vi "lorentzian from circle corners V6.vi"(6 "fragment  : cursor window":T4={"left"=2378.60310421286, "right "=2421.6740576496672, "center"=2421.6740576496672, "window"=2421.6740576496672, "cursors"=[], "relative"=0, "absolute"=0, "plot ref"=refnum, "Cursor List"=[], "fixed vertical offset"=2421.6740576496672, "vertical offset"=2421.6740576496672, "horizontal offset"=2421.6740576496672, "default window frac"=2421.6740576496672, "kind"=enum."symmetric"}, 7 "update z(inf)":enum16{"update z(inf)", "do not update z(inf)"}(ring)=enum."do not update z(inf)", 8 "omega map rameters in":T6={"map method"=enum."less trivial", "2:window factor"=1, "left"=3.0, "right"=3.0, "omega"=3.0, "gamma"=3.0, "theta0"=3.0, "use points"=enum."decimated", "z(inf) method"=enum."median"}, 9 "main VI  path":path, 10 "parameters in: center detection":T3={"number of 2D grid points"=200, "# of points in pond"=93, "# of points in window"=4107, "decimation threshold"=1, "normalization factor"=0.005102552585135461, "pond scale factor "=3.0, "normalized z"=[], "decimated z"=[], "decimated omega"=[], "omega in window"=[], "z in window"=[], "data center"=-0.0014901433980738042-0.0014987103874714112i, "inverse"=[], "linear "=[], "omega around"=[], "phase around center"=[], "fit for phase around senter "=[], "three points"={[], []}}, 11 "lorentzian in":T1={"Amplitude"=-1.0311345636926572, "omega(0)"=-1.0311345636926572, "Gamma"=-1.0311345636926572, "phase"=-1.0311345636926572, "Q"=-1.0311345636926572, "Norm  Ampl"=-1.0311345636926572, "z (inf)"=-1.0311345636926572+0.0i, "4corners"={"z (-pi/2)"=-1.0311345636926572+0.5736824521422934i, "z(inf)"=-0.5200164984937075+1.0975277942502903i, "z (pi/2)"=-1.0311345636926572+0.5736824521422934i, "z center"=-0.5136528600391839+0.580046090596817i, "z(0)"=-0.5200164984937075+1.0975277942502903i, "radius"=-1.0311345636926572}} {"Q" format="%#_8f"; "phase" format="%#_6f"; "Gamma" format="%#_8f"; "omega(0)" format="%#_8f"}) -> (0 "omega map parameters  out":T6={"map method"=enum."less trivial", "2:window factor"=1, "left"=3.0, "right"=3.0, "omega"=3.0, "gamma"=3.0, "theta0"=3.0, "use points"=enum."decimated", "z(inf) method"=enum."median"}, 2 "parameters out  : center detection":T3={"number of 2D grid points"=200, "# of points in pond"=93, "# of points in window"=4107, "decimation threshold"=1, "normalization factor"=0.005102552585135461, "pond scale factor "=3.0, "normalized z"=[], "decimated z"=[], "decimated omega"=[], "omega in window"=[], "z in window"=[], "data center"=-0.0014901433980738042-0.0014987103874714112i, "inverse"=[], "linear "=[], "omega around"=[], "phase around center"=[], "fit for phase around senter "=[], "three points"={[], []}}, 3 "lorentzian out":T1={"Amplitude"=-1.0311345636926572, "omega(0)"=-1.0311345636926572, "Gamma"=-1.0311345636926572, "phase"=-1.0311345636926572, "Q"=-1.0311345636926572, "Norm  Ampl"=-1.0311345636926572, "z (inf)"=-1.0311345636926572+0.0i, "4corners"={"z (-pi/2)"=-1.0311345636926572+0.5736824521422934i, "z(inf)"=-0.5200164984937075+1.0975277942502903i, "z (pi/2)"=-1.0311345636926572+0.5736824521422934i, "z center"=-0.5136528600391839+0.580046090596817i, "z(0)"=-0.5200164984937075+1.0975277942502903i, "radius"=-1.0311345636926572}} {"Q" format="%#_8f"; "phase" format="%#_6f"; "Gamma" format="%#_8f"; "omega(0)" format="%#_8f"})   [LabVIEW 2010]
uses:
  lorentzian.ctl
  circle corners.ctl
  omega map parameters.ctl
  single fit parameters.ctl
  cursor winow.ctl
  <vilib>/Utility/miscctls.llb/LVCursorListTypeDef.ctl
  <vilib>/gmath/NumericalOptimization/LM model function reference.ctl
  <vilib>/Analysis/6fits.llb/Curve Fitting Criteria.ctl
  <vilib>/Analysis/baseanly.llb/Mean.vi
  <vilib>/Analysis/baseanly.llb/Median.vi
  <vilib>/gmath/NumericalOptimization/Nonlinear Curve Fit LM.vi
  <vilib>/Analysis/NI_AALPro.lvlib
  <vilib>/gmath/NI_Gmath.lvlib
  <vilib>/gmath/NumericalOptimization/Nonlinear Curve Fit LM formula string.vi
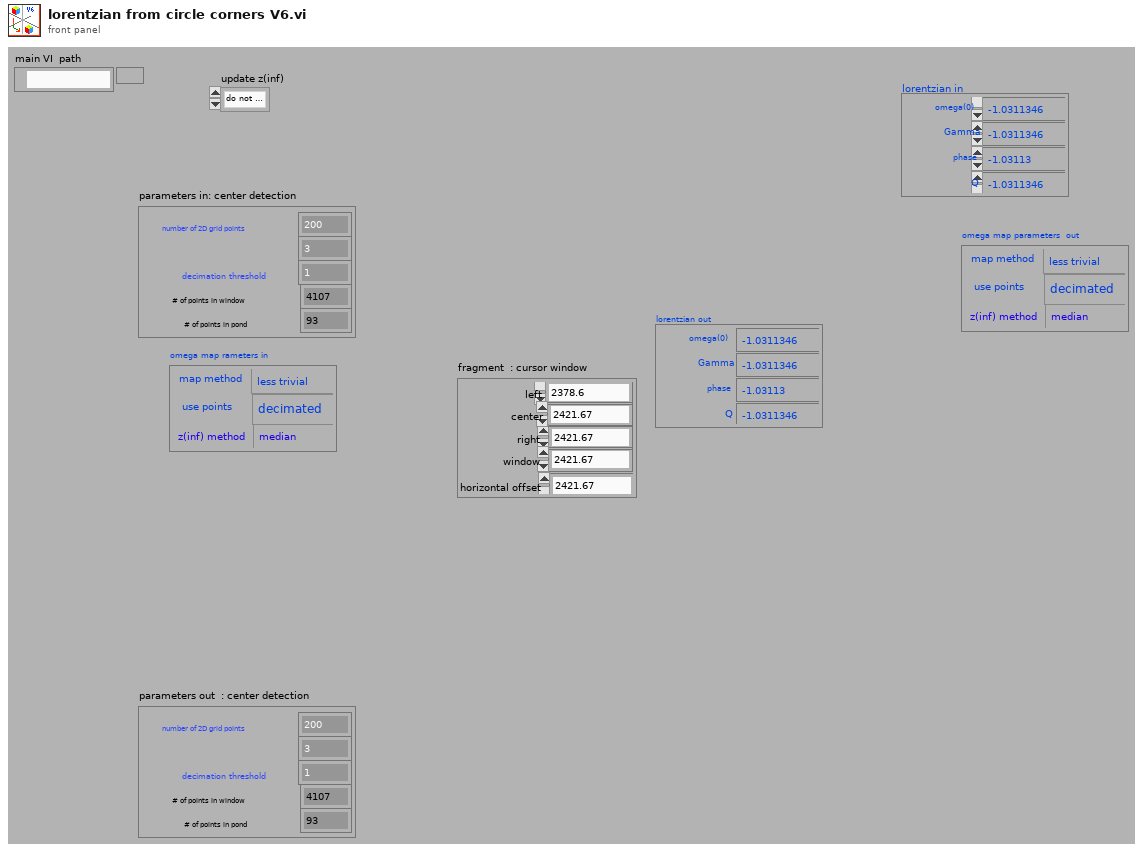
[diagram p1: front panel]
types:
  T1 = typedef "lorentzian.ctl" = cluster{"Amplitude":dbl, "omega(0)":dbl, "Gamma":dbl, "phase":dbl, "Q":dbl, "Norm  Ampl":dbl, "z (inf)":cdb, "4corners":T2}
  T2 = typedef "circle corners.ctl" = cluster{"z (-pi/2)":cdb, "z(inf)":cdb, "z (pi/2)":cdb, "z center":cdb, "z(0)":cdb, "radius":dbl}
  T3 = typedef "single fit parameters.ctl" = cluster{"number of 2D grid points":i32, "# of points in pond":i32, "# of points in window":i32, "decimation threshold":i32, "normalization factor":dbl, "pond scale factor ":dbl, "normalized z":cdb[], "decimated z":cdb[], "decimated omega":dbl[], "omega in window":dbl[], "z in window":cdb[], "data center":cdb, "inverse":cdb[], "linear ":cdb[], "omega around":dbl[], "phase around center":dbl[], "fit for phase around senter ":dbl[], "three points":cluster{dbl[], dbl[]}}
  T4 = typedef "cursor winow.ctl" = cluster{"left":dbl, "right ":dbl, "center":dbl, "window":dbl, "cursors":i32[], "relative":i32, "absolute":i32, "plot ref":refnum<vi>, "Cursor List":T5, "fixed vertical offset":dbl, "vertical offset":dbl, "horizontal offset":dbl, "default window frac":dbl, "kind":enum16{"symmetric", "skewed", "fancy"}}
  T5 = typedef "LVCursorListTypeDef.ctl" = cluster{"Name":string, "Color":u32, "Style":u8, "Point Style":u8, "Name Visible":bool, "Allow Drag":bool, "Cursor Mode":u32, "Plot":i32, "Index":i32, "Position":cluster{"X":dbl, "Y":dbl}, "X Scale":u32, "Y Scale":u32, "Watch Plots":i32[], "Watch All Plots":bool, "Plot Area":i32, "Label Offset":cluster{"X":dbl, "Y":dbl}}[]
  T6 = typedef "omega map parameters.ctl" = cluster{"map method":enum16{"simple", "less trivial", "around center", "geometry"}, "2:window factor":i32, "left":dbl, "right":dbl, "omega":dbl, "gamma":dbl, "theta0":dbl, "use points":enum16{"all in window", "decimated"}, "z(inf) method":enum16{"median", "method 2", "histogram"}}
  T7 = enum16{"simple", "less trivial", "around center", "geometry"}
  T8 = typedef "NI_Gmath.lvlib/LM model function reference.ctl" = refnum<vi>
  T9 = cluster{"model":string, "Parameters":string[], "x":string}
  T10 = typedef "NI_AALPro.lvlib/Curve Fitting Criteria.ctl" = u16
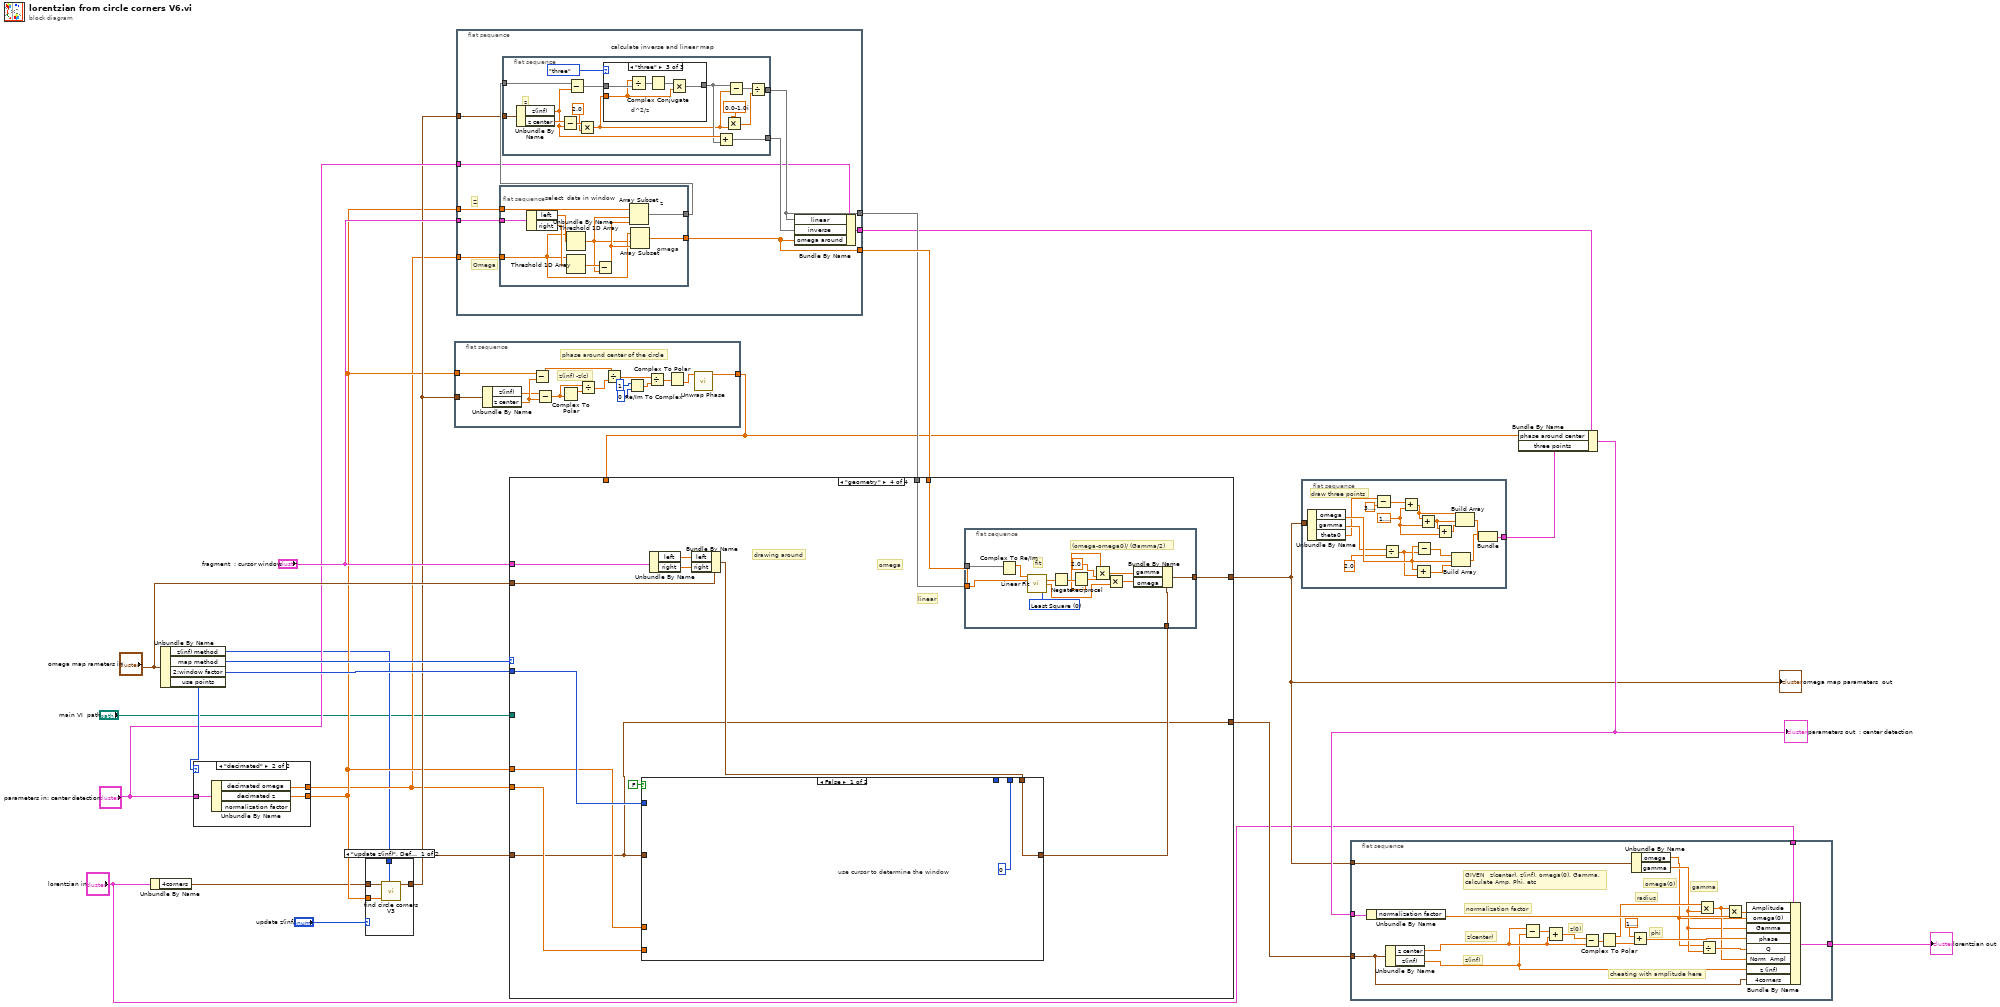
[diagram p0: block diagram]
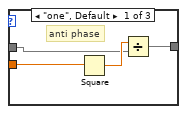
[diagram p2: hidden frame]
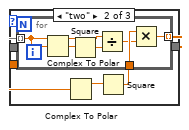
[diagram p3: hidden frame]
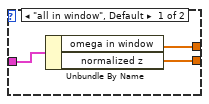
[diagram p5: hidden frame]
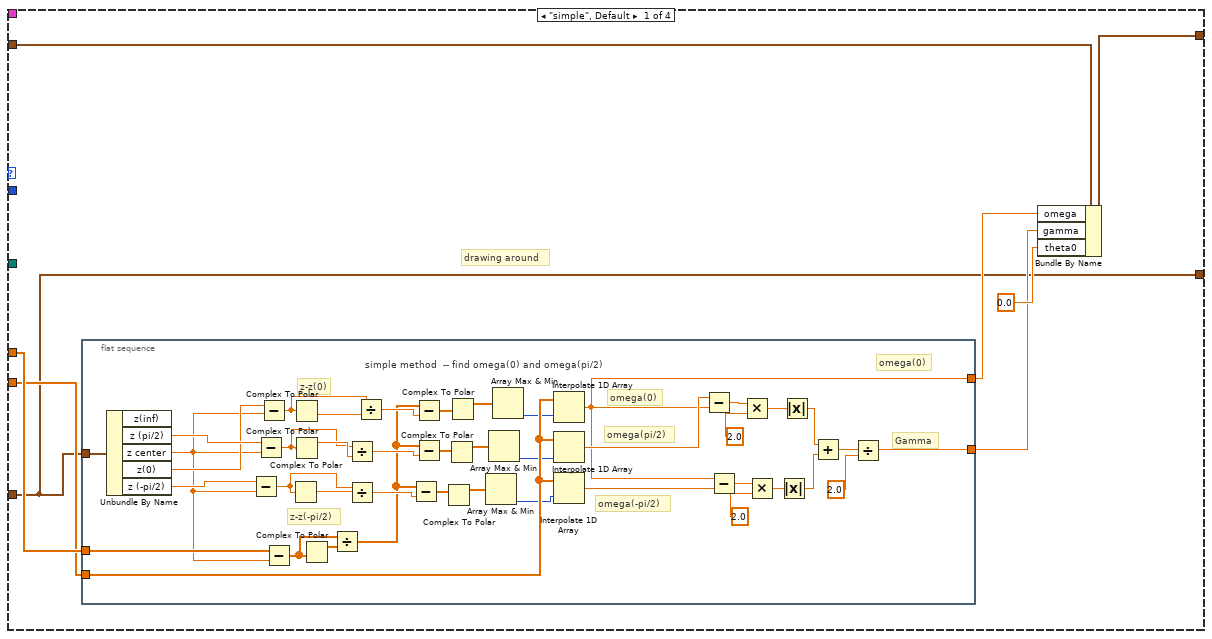
[diagram p6: hidden frame]
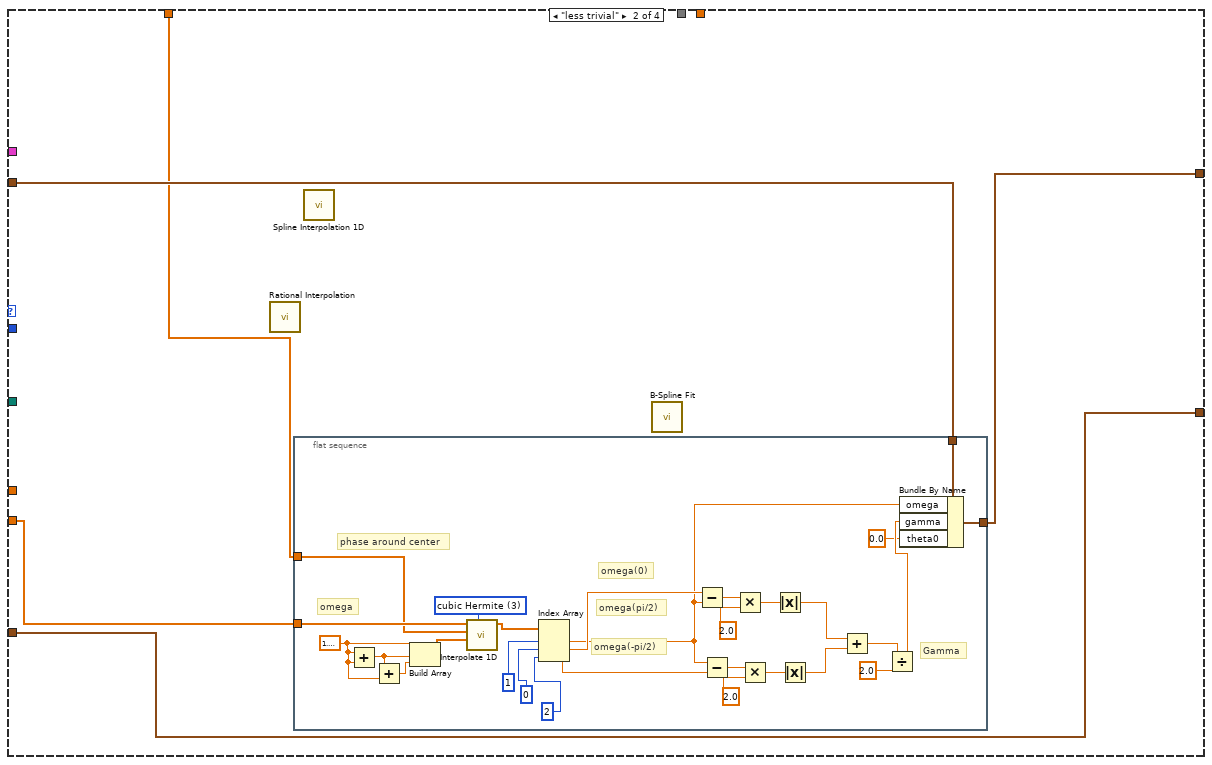
[diagram p7: hidden frame]
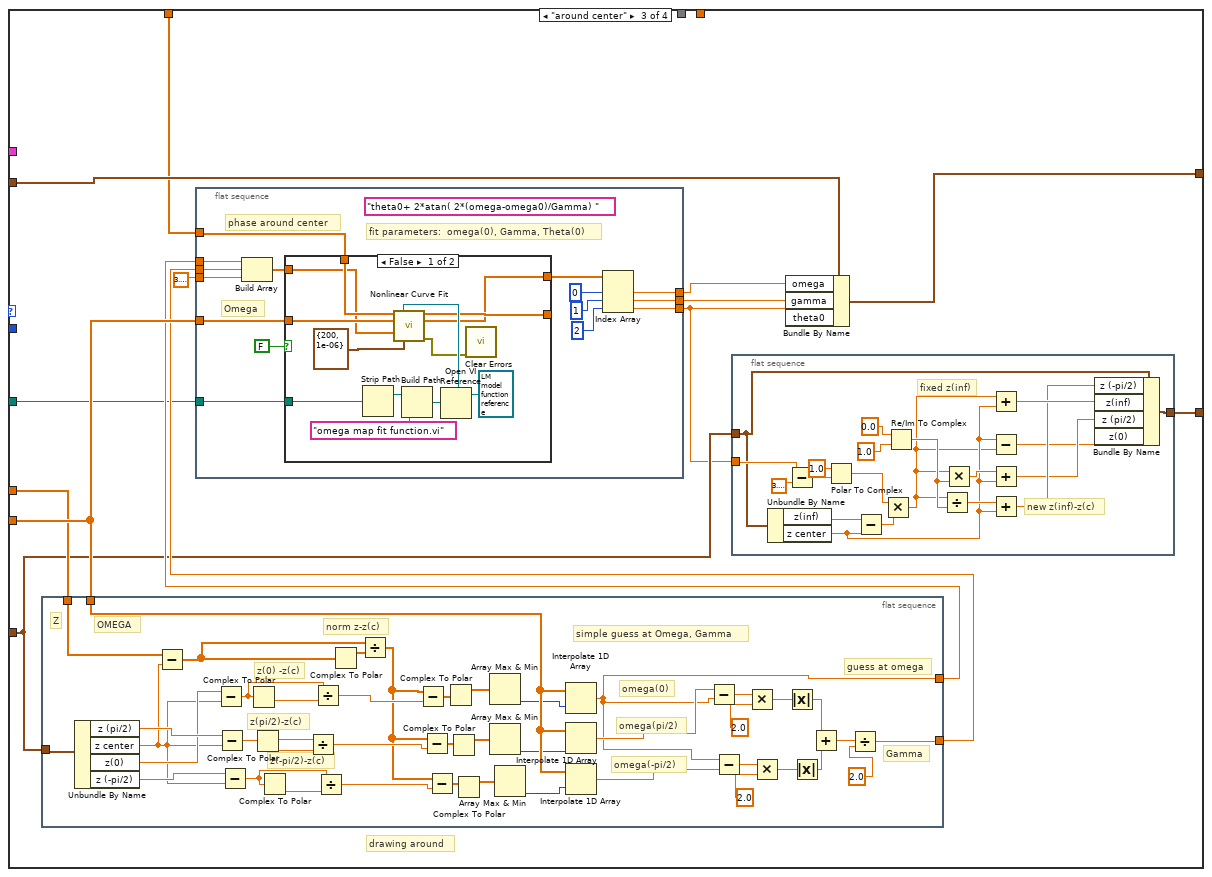
[diagram p8: hidden frame]
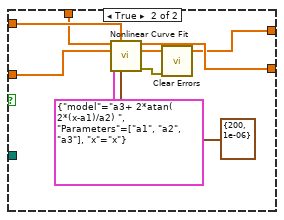
[diagram p9: hidden frame]
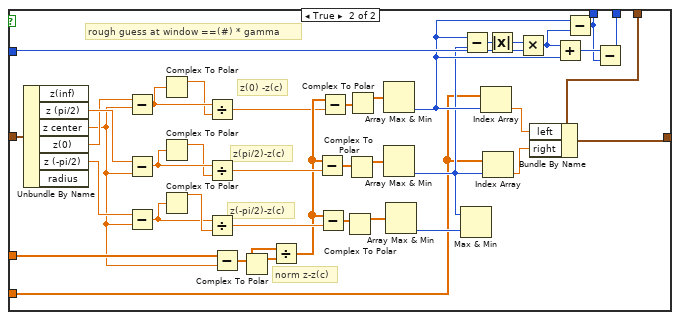
[diagram p10: hidden frame]
diagram:
  n1 = Unbundle By Name("lorentzian in") -> ("4corners"=w3:T2)
  n2 = Unbundle By Name("omega map rameters in") -> ("z(inf) method"=w4:enum16{"median", "method 2", "histogram"}, "map method"=w23:T7, "2:window factor"=w21:i32, "use points"=w20:enum16{"all in window", "decimated"})
  n3 = case shown="\"decimated\"" w20 {
    tunnel: "parameters in: center detection" -> [w26 w29]
    tunnel: [w25 w28] -> w11
    tunnel: [w24 w27] -> w13
    frame "all in window", Default {
      n4 = Unbundle By Name(w26) -> ("omega in window"=w25:dbl[], "normalized z"=w24:cdb[])
    }
    frame "decimated" {
      n5 = Unbundle By Name(w29) -> ("decimated omega"=w28:dbl[], "decimated z"=w27:cdb[])  [unwired: 1 out]
    }
  }
  n6 = case shown="\"update z(inf)\", Default" "update z(inf)" {
    tunnel: [w32 w34] -> w14
    tunnel: w3 -> [w33 w34]
    tunnel: w13 -> [w31 _]
    tunnel: w4 -> [w30 _]
    frame "update z(inf)", Default {
      n7 = call "find circle corners V3.vi"("method"=w30, "z"=w31, "circle corners in"=w33) -> ("circle corners out"=w32:T2)  [unwired: 8 in]
    }
    frame "do not update z(inf)" {
    }
  }
  n8 = flat-sequence {
    tunnel: w14 -> [w37]
    tunnel: w13 -> [w36]
    tunnel: [w35] -> w9
    frame #0 {
      # "phase around center of the circle"
      # "z(inf) -z(c)"
      n9 = Unbundle By Name(w37) -> ("z(inf)"=w39:cdb, "z center"=w40:cdb)
      n10 = Subtract(x=w36, y=w40) -> (x-y=w48:cdb[])
      n11 = Subtract(x=w39, y=w40) -> (x-y=w38:cdb)
      n12 = Complex To Polar(r * e^(i*theta)=w38) -> (r=w49:dbl)  [unwired: 1 out]
      n13 = Divide(x=w38, y=w49) -> (x/y=w41:cdb)
      n14 = Divide(x=w48, y=w41) -> (x/y=w44:cdb[])
      n15 = Re/Im To Complex(1:0, 2:1) -> (0:w46:cdb)
      n16 = Divide(x=w44, y=w46) -> (x/y=w47:cdb[])
      n17 = Complex To Polar(r * e^(i*theta)=w47) -> (theta=w42:dbl[])  [unwired: 1 out]
      n18 = call <vilib>:"Unwrap Phase.vi"("Phase"=w42) -> ("Unwrapped Phase"=w35:dbl[])  [unwired: 9 in, 1 out]
    }
  }
  n19 = flat-sequence {
    tunnel: [w57] -> w18
    tunnel: w14 -> [w56]
    tunnel: w13 -> [w55]
    tunnel: "fragment  : cursor window" -> [w54]
    tunnel: w11 -> [w53]
    tunnel: [w52] -> w10
    tunnel: [w51] -> w16
    tunnel: "parameters in: center detection" -> [w50]
    frame #0 {
      # "calculate inverse and linear map"
      # "Z"
      # "Omega"
      n20 = flat-sequence {
        tunnel: [w100] -> w58
        tunnel: [w99] -> w57
        tunnel: w55 -> [w98]
        tunnel: w54 -> [w97]
        tunnel: w53 -> [w96]
        frame #0 {
          # "select  data in window"
          # "omega"
          # "z"
          n21 = Unbundle By Name(w97) -> ("left"=w101:dbl, "right"=w102:dbl)
          n22 = Threshold 1D Array(2:w101, 3:w96) -> (0:w95:dbl)  [unwired: 1 in]
          n23 = Threshold 1D Array(2:w102, 3:w96) -> (0:w103:dbl)  [unwired: 1 in]
          n24 = Subtract(x=w103, y=w95) -> (x-y=w104:dbl)
          n25 = Array Subset(array=w98, index=w95, length=w104) -> (w100:cdb[])
          n26 = Array Subset(array=w96, index=w95, length=w104) -> (w99:dbl[])
        }
      }
      n27 = flat-sequence {
        tunnel: [w74] -> w59
        tunnel: w58 -> [w69]
        tunnel: w56 -> [w63]
        tunnel: [w62] -> w51
        frame #0 {
          # "z"
          n28 = Unbundle By Name(w63) -> ("z(inf)"=w72:cdb, "z center"=w73:cdb)
          n29 = Subtract(x=w73, y=w72) -> (x-y=w65:cdb)
          n30 = Subtract(x=w69, y=w72) -> (x-y=w66:cdb[])
          n31 = Multiply(x=w65, y=2.0) -> (x*y=w61:cdb)
          n32 = case shown="\"three\"" enum16{"one", "three", "two"}."three" {
            tunnel: w66 -> [w76 w83 w94]
            tunnel: [w75 w80 w90] -> w67
            tunnel: w61 -> [w78 w79 w91]
            frame "one", Default {
              # "anti phase"
              n33 = Square(x=w78) -> (x^2=w77:cdb)
              n34 = Divide(x=w77, y=w76) -> (x/y=w75:cdb[])
            }
            frame "two" {
              n35 = Complex To Polar(r * e^(i*theta)=w79) -> (r=w82:dbl)  [unwired: 1 out]
              n36 = Square(x=w82) -> (x^2=w81:dbl)
              n37 = for {
                tunnel: w83 -> [w89] mode=indexing
                tunnel: w81 -> [w86]
                tunnel: [w84] -> w80 mode=indexing
                n38 = Complex To Polar(r * e^(i*theta)=w89) -> (r=w87:dbl)  [unwired: 1 out]
                n39 = Square(x=w87) -> (x^2=w88:dbl)
                n40 = Divide(x=w89, y=w88) -> (x/y=w85:cdb)
                n41 = Multiply(x=w86, y=w85) -> (x*y=w84:cdb)
              }
            }
            frame "three" {
              # "d^2/z"
              n42 = Divide(x=w91, y=w94) -> (x/y=w93:cdb[])
              n43 = Complex Conjugate(1:w93) -> (0:w92:cdb[])
              n44 = Multiply(x=w92, y=w91) -> (x*y=w90:cdb[])
            }
          }
          n45 = Add(x=w72, y=w67) -> (x+y=w74:cdb[])
          n46 = Multiply(x=cdb 0.0-1.0i ("y"), y=w61) -> (x*y=w70:cdb)
          n47 = Subtract(x=w67, y=w61) -> (x-y=w68:cdb[])
          n48 = Divide(x=w68, y=w70) -> (x/y=w62:cdb[])
        }
      }
      n49 = Bundle By Name(cluster=w50, "linear"=w51, "inverse"=w59, "omega around"=w57) -> (w52:T3)
    }
  }
  n50 = case shown="\"geometry\"" w23 {
    tunnel: w14 -> [w105 w155 w192 w300]
    tunnel: w13 -> [w112 _ w193 w311]
    tunnel: w11 -> [w111 w157 w200 w302]
    tunnel: "omega map rameters in" -> [w109 w159 w199 w309]
    tunnel: [w108 w158 w201 w313] -> w6
    tunnel: w21 -> [_ _ _ w312]
    tunnel: "fragment  : cursor window" -> [_ _ _ w304]
    tunnel: w18 -> [_ _ _ w303]
    tunnel: w16 -> [_ _ _ w301]
    tunnel: w9 -> [_ w156 w191 _]
    tunnel: [w105 w155 w189 w300] -> w5
    tunnel: "main VI  path" -> [_ _ w188 _]
    frame "simple", Default {
      # "drawing around"
      n51 = flat-sequence {
        tunnel: w105 -> [w150]
        tunnel: w112 -> [w149]
        tunnel: w111 -> [w138]
        tunnel: [w115] -> w107
        tunnel: [w114] -> w106
        frame #0 {
          # "simple method  -- find omega(0) and omega(pi/2)"
          # "omega(0)"
          # "z-z(-pi/2)"
          # "z-z(0)"
          # "omega(-pi/2)"
          # "omega(pi/2)"
          # "omega(0)"
          # "Gamma"
          n52 = Unbundle By Name(w150) -> ("z (pi/2)"=w148:cdb, "z center"=w113:cdb, "z(0)"=w147:cdb, "z (-pi/2)"=w146:cdb)  [unwired: 1 out]
          n53 = Subtract(x=w146, y=w113) -> (x-y=w133:cdb)
          n54 = Subtract(x=w148, y=w113) -> (x-y=w132:cdb)
          n55 = Subtract(x=w147, y=w113) -> (x-y=w137:cdb)
          n56 = Subtract(x=w149, y=w113) -> (x-y=w130:cdb[])
          n57 = Complex To Polar(r * e^(i*theta)=w133) -> (r=w135:dbl)  [unwired: 1 out]
          n58 = Complex To Polar(r * e^(i*theta)=w137) -> (r=w136:dbl)  [unwired: 1 out]
          n59 = Complex To Polar(r * e^(i*theta)=w132) -> (r=w134:dbl)  [unwired: 1 out]
          n60 = Complex To Polar(r * e^(i*theta)=w130) -> (r=w131:dbl[])  [unwired: 1 out]
          n61 = Divide(x=w130, y=w131) -> (x/y=w126:cdb[])
          n62 = Divide(x=w132, y=w134) -> (x/y=w128:cdb)
          n63 = Divide(x=w133, y=w135) -> (x/y=w127:cdb)
          n64 = Divide(x=w137, y=w136) -> (x/y=w129:cdb)
          n65 = Subtract(x=w126, y=w127) -> (x-y=w124:cdb[])
          n66 = Subtract(x=w126, y=w129) -> (x-y=w125:cdb[])
          n67 = Subtract(x=w126, y=w128) -> (x-y=w123:cdb[])
          n68 = Complex To Polar(r * e^(i*theta)=w124) -> (r=w120:dbl[])  [unwired: 1 out]
          n69 = Complex To Polar(r * e^(i*theta)=w123) -> (r=w121:dbl[])  [unwired: 1 out]
          n70 = Complex To Polar(r * e^(i*theta)=w125) -> (r=w122:dbl[])  [unwired: 1 out]
          n71 = Array Max & Min(array=w120) -> (min index (indices)=w119:i32)  [unwired: 3 out]
          n72 = Array Max & Min(array=w121) -> (min index (indices)=w118:i32)  [unwired: 3 out]
          n73 = Array Max & Min(array=w122) -> (min index (indices)=w117:i32)  [unwired: 3 out]
          n74 = Interpolate 1D Array(1:w117, 2:w138) -> (0:w115:dbl)
          n75 = Interpolate 1D Array(1:w118, 2:w138) -> (0:w151:dbl)
          n76 = Interpolate 1D Array(1:w119, 2:w138) -> (0:w139:dbl)
          n77 = Subtract(x=w151, y=w115) -> (x-y=w154:dbl)
          n78 = Subtract(x=w115, y=w139) -> (x-y=w145:dbl)
          n79 = Multiply(x=w154, y=2.0) -> (x*y=w152:dbl)
          n80 = Multiply(x=w145, y=2.0) -> (x*y=w143:dbl)
          n81 = Absolute Value(x=w143) -> (abs(x)=w116:dbl)
          n82 = Absolute Value(x=w152) -> (abs(x)=w142:dbl)
          n83 = Add(x=w142, y=w116) -> (x+y=w141:dbl)
          n84 = Divide(x=w141, y=2.0) -> (x/y=w114:dbl)
        }
      }
      n85 = Bundle By Name(cluster=w109, "omega"=w107, "gamma"=w106, "theta0"=0.0 ("phi0")) -> (w108:T6)
    }
    frame "less trivial" {
      n86 = call <vilib>:"Rational Interpolation.vi"() -> ()  [unwired: 3 in, 3 out]
      n87 = flat-sequence {
        tunnel: w159 -> [w166]
        tunnel: [w165] -> w158
        tunnel: w157 -> [w162]
        tunnel: w156 -> [w161]
        frame #0 {
          w175 = 1.5707963267948966
          w177 = 3 items=["nearest", "linear", "spline", "cubic Hermite", "Lagrange"] ("method")
          # "phase around center"
          # "omega"
          # "omega(-pi/2)"
          # "omega(pi/2)"
          # "omega(0)"
          # "Gamma"
          n88 = Add(x=w175, y=w175) -> (x+y=w176:dbl)
          n89 = Add(x=w176, y=w175) -> (x+y=w174:dbl)
          n90 = Build Array(w175, w176, w174) -> (w173:dbl[])
          n91 = call <vilib>:"Interpolate 1D.vi"("method"=w177, "xi"=w173, "X"=w161, "Y"=w162) -> ("yi"=w169:dbl[])  [unwired: 5 in, 2 out]
          n92 = Index Array(array=w169, index #1=1, index #2=0, index #3=2) -> (element #1=w164:dbl, element #2=w168:dbl, element #3=w167:dbl)
          n93 = Subtract(x=w168, y=w164) -> (x-y=w187:dbl)
          n94 = Subtract(x=w164, y=w167) -> (x-y=w184:dbl)
          n95 = Multiply(x=w187, y=2.0) -> (x*y=w185:dbl)
          n96 = Multiply(x=w184, y=2.0) -> (x*y=w182:dbl)
          n97 = Absolute Value(x=w185) -> (abs(x)=w181:dbl)
          n98 = Absolute Value(x=w182) -> (abs(x)=w178:dbl)
          n99 = Add(x=w181, y=w178) -> (x+y=w180:dbl)
          n100 = Divide(x=w180, y=2.0) -> (x/y=w163:dbl)
          n101 = Bundle By Name(cluster=w166, "omega"=w164, "gamma"=w163, "theta0"=0.0 ("phi0")) -> (w165:T6)
        }
      }
      n102 = call <vilib>:"Spline Interpolation 1D.vi"() -> ()  [unwired: 9 in, 3 out]
      n103 = call <vilib>:"B-Spline Fit.vi"() -> ()  [unwired: 12 in, 4 out]
    }
    frame "around center" {
      # "drawing around"
      n104 = flat-sequence {
        tunnel: w200 -> [w299]
        tunnel: [w267] -> w195
        tunnel: [w264] -> w194
        tunnel: w192 -> [w263]
        tunnel: w193 -> [w261]
        frame #0 {
          # "guess at omega"
          # "simple guess at Omega, Gamma"
          # "OMEGA"
          # "Z"
          # "norm z-z(c)"
          # "omega(-pi/2)"
          # "omega(pi/2)"
          # "omega(0)"
          # "Gamma"
          # "z(pi/2)-z(c)"
          # "z(-pi/2)-z(c)"
          # "z(0) -z(c)"
          n105 = Unbundle By Name(w263) -> ("z (pi/2)"=w298:cdb, "z center"=w262:cdb, "z(0)"=w297:cdb, "z (-pi/2)"=w296:cdb)
          n106 = Subtract(x=w261, y=w262) -> (x-y=w259:cdb[])
          n107 = Subtract(x=w297, y=w262) -> (x-y=w295:cdb)
          n108 = Subtract(x=w298, y=w262) -> (x-y=w291:cdb)
          n109 = Subtract(x=w296, y=w262) -> (x-y=w292:cdb)
          n110 = Complex To Polar(r * e^(i*theta)=w295) -> (r=w294:dbl)  [unwired: 1 out]
          n111 = Complex To Polar(r * e^(i*theta)=w291) -> (r=w281:dbl)  [unwired: 1 out]
          n112 = Complex To Polar(r * e^(i*theta)=w292) -> (r=w293:dbl)  [unwired: 1 out]
          n113 = Divide(x=w291, y=w281) -> (x/y=w289:cdb)
          n114 = Divide(x=w295, y=w294) -> (x/y=w290:cdb)
          n115 = Divide(x=w292, y=w293) -> (x/y=w288:cdb)
          n116 = Complex To Polar(r * e^(i*theta)=w259) -> (r=w260:dbl[])  [unwired: 1 out]
          n117 = Divide(x=w259, y=w260) -> (x/y=w258:cdb[])
          n118 = Subtract(x=w258, y=w290) -> (x-y=w287:cdb[])
          n119 = Subtract(x=w258, y=w289) -> (x-y=w285:cdb[])
          n120 = Subtract(x=w258, y=w288) -> (x-y=w286:cdb[])
          n121 = Complex To Polar(r * e^(i*theta)=w287) -> (r=w284:dbl[])  [unwired: 1 out]
          n122 = Complex To Polar(r * e^(i*theta)=w285) -> (r=w283:dbl[])  [unwired: 1 out]
          n123 = Complex To Polar(r * e^(i*theta)=w286) -> (r=w282:dbl[])  [unwired: 1 out]
          n124 = Array Max & Min(array=w284) -> (min index (indices)=w270:i32)  [unwired: 3 out]
          n125 = Array Max & Min(array=w283) -> (min index (indices)=w269:i32)  [unwired: 3 out]
          n126 = Array Max & Min(array=w282) -> (min index (indices)=w268:i32)  [unwired: 3 out]
          n127 = Interpolate 1D Array(1:w270, 2:w299) -> (0:w264:dbl)
          n128 = Interpolate 1D Array(1:w269, 2:w299) -> (0:w266:dbl)
          n129 = Interpolate 1D Array(1:w268, 2:w299) -> (0:w265:dbl)
          n130 = Subtract(x=w266, y=w264) -> (x-y=w280:dbl)
          n131 = Subtract(x=w264, y=w265) -> (x-y=w277:dbl)
          n132 = Multiply(x=w280, y=2.0) -> (x*y=w278:dbl)
          n133 = Multiply(x=w277, y=2.0) -> (x*y=w275:dbl)
          n134 = Absolute Value(x=w278) -> (abs(x)=w274:dbl)
          n135 = Absolute Value(x=w275) -> (abs(x)=w271:dbl)
          n136 = Add(x=w274, y=w271) -> (x+y=w273:dbl)
          n137 = Divide(x=w273, y=2.0) -> (x/y=w267:dbl)
        }
      }
      n138 = flat-sequence {
        tunnel: w200 -> [w236]
        tunnel: [w235] -> w198
        tunnel: [w234] -> w197
        tunnel: 3.141592653589793 -> [w233]
        tunnel: w195 -> [w231]
        tunnel: w194 -> [w230]
        tunnel: [w225] -> w190
        tunnel: w191 -> [w223]
        tunnel: w188 -> [w222]
        frame #0 {
          (unwired) "theta0+ 2*atan( 2*(omega-omega0)/Gamma) " ("model")
          # "phase around center"
          # "Omega"
          # "fit parameters:  omega(0), Gamma, Theta(0)"
          n139 = Build Array(w230, w231, w233) -> (w232:dbl[])
          n140 = case shown="False" FALSE {
            tunnel: w236 -> [w241 w257]
            tunnel: w232 -> [w240 w256]
            tunnel: [w239 w255] -> _
            tunnel: w223 -> [w242 w254]
            tunnel: [w238 w253] -> w229
            tunnel: w222 -> [w237 _]
            frame False {
              n141 = Strip Path(path=w237) -> (stripped path=w248:path)  [unwired: 1 out]
              n142 = Build Path(base path=w248, name or relative path="omega map fit function.vi" ("f(x,a) VI name Complex")) -> (appended path=w246:path)
              n143 = Open VI Reference(type specifier VI Refnum (for type only)=T8 refnum ("f(x,a)"), vi path=w246) -> (vi reference=w245:T8)  [unwired: 1 in, 4 out]
              n144 = call-poly <vilib>:"Nonlinear Curve Fit.vi"("Y"=w242, "f(x,a)"=w245, "X"=w241, "initial parameters"=w240, "termination"=cluster{"max iteration":i32, "tolerance":dbl} {"max iteration"=200, "tolerance"=1e-06}) -> ("best nonlinear fit"=w239:dbl[], "best fit parameters"=w238:dbl[], "error out"=w243:errorcluster)  [unwired: 5 in, 3 out]
              n145 = call <vilib>:"Clear Errors.vi"("error in (no error)"=w243) -> ()  [unwired: 6 in, 1 out]
            }
            frame True {
              n146 = call-poly <vilib>:"Nonlinear Curve Fit.vi"("Y"=w254, "initial parameters"=w256, "X"=w257, "model description"=T9 {"model"="a3+ 2*atan( 2*(x-a1)/a2) ", "Parameters"=["a1", "a2", "a3"], "x"="x"}, "termination"=cluster{"max iteration":i32, "tolerance":dbl} {"max iteration"=200, "tolerance"=1e-06}) -> ("best nonlinear fit"=w255:dbl[], "best fit parameters"=w253:dbl[], "error out"=w250:errorcluster)  [unwired: 6 in, 2 out]
              n147 = call <vilib>:"Clear Errors.vi"("error in (no error)"=w250) -> ()  [unwired: 6 in, 1 out]
            }
          }
          n148 = Index Array(array=w229, index #1=0, index #2=1, index #3=2) -> (element #1=w235:dbl, element #2=w234:dbl, element #3=w225:dbl)
        }
      }
      n149 = flat-sequence {
        tunnel: w192 -> [w203]
        tunnel: w190 -> [w218]
        tunnel: [w202] -> w189
        frame #0 {
          # "new z(inf)-z(c)"
          # "fixed z(inf)"
          n150 = Unbundle By Name(w203) -> ("z(inf)"=w220:cdb, "z center"=w205:cdb)
          n151 = Subtract(x=w218, y=3.141592653589793) -> (x-y=w217:dbl)
          n152 = Polar To Complex(1:w217, 2:1.0 ("r")) -> (0:w215:cdb)
          n153 = Subtract(x=w220, y=w205) -> (x-y=w219:cdb)
          n154 = Multiply(x=w215, y=w219) -> (x*y=w204:cdb)
          n155 = Re/Im To Complex(1:1.0 ("y"), 2:0.0 ("x")) -> (0:w210:cdb)
          n156 = Divide(x=w204, y=w210) -> (x/y=w211:cdb)
          n157 = Multiply(x=w204, y=w210) -> (x*y=w212:cdb)
          n158 = Add(x=w204, y=w205) -> (x+y=w209:cdb)
          n159 = Subtract(x=w205, y=w204) -> (x-y=w206:cdb)
          n160 = Add(x=w212, y=w205) -> (x+y=w207:cdb)
          n161 = Add(x=w211, y=w205) -> (x+y=w208:cdb)
          n162 = Bundle By Name(cluster=w203, "z (-pi/2)"=w208, "z(inf)"=w209, "z (pi/2)"=w207, "z(0)"=w206) -> (w202:T2)
        }
      }
      n163 = Bundle By Name(cluster=w199, "omega"=w198, "gamma"=w197, "theta0"=w190) -> (w201:T6)
    }
    frame "geometry" {
      # "omega"
      # "linear"
      # "drawing around"
      n164 = Unbundle By Name(w304) -> ("left"=w306:dbl, "right"=w305:dbl)
      n165 = Bundle By Name(cluster=w309, "left"=w306, "right"=w305) -> (w308:T6)
      n166 = case shown="False" FALSE {
        tunnel: w312 -> [_ w343]
        tunnel: w311 -> [_ w342]
        tunnel: [w327 w341] -> _
        tunnel: [w327 w340] -> _
        tunnel: w302 -> [_ w337]
        tunnel: w300 -> [_ w335]
        tunnel: [w328 w331] -> w307
        tunnel: w308 -> [w328 w330]
        frame False {
          w327 = 0
          # "use cursor to determine the window"
        }
        frame True {
          # "rough guess at window ==(#) * gamma"
          # "z(pi/2)-z(c)"
          # "norm z-z(c)"
          # "z(-pi/2)-z(c)"
          # "z(0) -z(c)"
          n167 = Unbundle By Name(w335) -> ("z (pi/2)"=w367:cdb, "z center"=w334:cdb, "z(0)"=w366:cdb, "z (-pi/2)"=w336:cdb)  [unwired: 2 out]
          n168 = Subtract(x=w366, y=w334) -> (x-y=w365:cdb)
          n169 = Subtract(x=w367, y=w334) -> (x-y=w361:cdb)
          n170 = Subtract(x=w336, y=w334) -> (x-y=w362:cdb)
          n171 = Complex To Polar(r * e^(i*theta)=w365) -> (r=w364:dbl)  [unwired: 1 out]
          n172 = Complex To Polar(r * e^(i*theta)=w361) -> (r=w349:dbl)  [unwired: 1 out]
          n173 = Complex To Polar(r * e^(i*theta)=w362) -> (r=w363:dbl)  [unwired: 1 out]
          n174 = Divide(x=w365, y=w364) -> (x/y=w329:cdb)
          n175 = Divide(x=w361, y=w349) -> (x/y=w359:cdb)
          n176 = Divide(x=w362, y=w363) -> (x/y=w358:cdb)
          n177 = Subtract(x=w342, y=w334) -> (x-y=w350:cdb[])
          n178 = Complex To Polar(r * e^(i*theta)=w350) -> (r=w360:dbl[])  [unwired: 1 out]
          n179 = Divide(x=w350, y=w360) -> (x/y=w351:cdb[])
          n180 = Subtract(x=w351, y=w359) -> (x-y=w355:cdb[])
          n181 = Subtract(x=w351, y=w358) -> (x-y=w356:cdb[])
          n182 = Subtract(x=w351, y=w329) -> (x-y=w357:cdb[])
          n183 = Complex To Polar(r * e^(i*theta)=w356) -> (r=w352:dbl[])  [unwired: 1 out]
          n184 = Complex To Polar(r * e^(i*theta)=w355) -> (r=w353:dbl[])  [unwired: 1 out]
          n185 = Complex To Polar(r * e^(i*theta)=w357) -> (r=w354:dbl[])  [unwired: 1 out]
          n186 = Array Max & Min(array=w354) -> (min index (indices)=w339:i32)  [unwired: 3 out]
          n187 = Array Max & Min(array=w353) -> (min index (indices)=w338:i32)  [unwired: 3 out]
          n188 = Array Max & Min(array=w352) -> (min index (indices)=w348:i32)  [unwired: 3 out]
          n189 = Max & Min(x=w338, y=w348) -> ()  [unwired: 2 out]
          n190 = Subtract(x=w339, y=w338) -> (x-y=w347:i32)
          n191 = Index Array(array=w337, index=w339) -> (element=w333:dbl)
          n192 = Index Array(array=w337, index=w338) -> (element=w332:dbl)
          n193 = Absolute Value(x=w347) -> (abs(x)=w346:i32)
          n194 = Multiply(x=w346, y=w343) -> (x*y=w345:i32)
          n195 = Bundle By Name(cluster=w330, "left"=w333, "right"=w332) -> (w331:T6)
          n196 = Add(x=w345, y=w339) -> (x+y=w344:i32)
          n197 = Subtract(x=w339, y=w345) -> (x-y=w340:i32)
          n198 = Subtract(x=w344, y=w340) -> (x-y=w341:i32)
        }
      }
      n199 = flat-sequence {
        tunnel: [w326] -> w313
        tunnel: w307 -> [w317]
        tunnel: w303 -> [w316]
        tunnel: w301 -> [w315]
        frame #0 {
          w325 = T10 0 items=["Least Square", "Least Absolute Residual", "Bisquare"] ("method")
          # "(omega-omega0)/ (Gamma/2)"
          # "fit"
          n200 = Complex To Re/Im(x + iy=w315) -> (x=w314:dbl[])  [unwired: 1 out]
          n201 = call <vilib>:"Linear Fit.vi"("Y"=w314, "X"=w316, "method"=w325) -> ("slope"=w323:dbl, "intercept"=w321:dbl)  [unwired: 8 in, 3 out]
          n202 = Negate(x=w323) -> (-x=w322:dbl)
          n203 = Reciprocal(x=w322) -> (1/x=w320:dbl)
          n204 = Multiply(x=w320, y=2.0) -> (x*y=w319:dbl)
          n205 = Multiply(x=w320, y=w321) -> (x*y=w318:dbl)
          n206 = Bundle By Name(cluster=w317, "gamma"=w319, "omega"=w318) -> (w326:T6)
        }
      }
    }
  }
  "omega map parameters  out" <- w6
  n207 = flat-sequence {
    tunnel: w6 -> [w384]
    tunnel: [w380] -> w8
    frame #0 {
      w372 = 1.5707963267948966
      # "draw three points"
      n208 = Unbundle By Name(w384) -> ("omega"=w383:dbl, "gamma"=w382:dbl, "theta0"=w381:dbl)
      n209 = Subtract(x=w381, y=3.141592653589793) -> (x-y=w368:dbl)
      n210 = Divide(x=w382, y=2.0) -> (x/y=w370:dbl)
      n211 = Add(x=w368, y=w372) -> (x+y=w373:dbl)
      n212 = Add(x=w383, y=w370) -> (x+y=w374:dbl)
      n213 = Subtract(x=w383, y=w370) -> (x-y=w375:dbl)
      n214 = Add(x=w373, y=w372) -> (x+y=w379:dbl)
      n215 = Add(x=w379, y=w372) -> (x+y=w378:dbl)
      n216 = Build Array(w375, w383, w374) -> (w376:dbl[])
      n217 = Build Array(w373, w379, w378) -> (w377:dbl[])
      n218 = Bundle(w376, w377) -> (w380:cluster{dbl[], dbl[]})  [unwired: 1 in]
    }
  }
  n219 = flat-sequence {
    tunnel: w5 -> [w385]
    tunnel: [w402] -> w12
    tunnel: w7 -> [w401]
    tunnel: w6 -> [w389]
    tunnel: "lorentzian in" -> [w386]
    frame #0 {
      # "GIVEN   z(center), z(inf), omega(0), Gamma, \ncalculate Amp, Phi, etc"
      # "z(center)"
      # "z(0)"
      # "z(inf)"
      # "normalization factor"
      # "radius"
      # "omega(0)"
      # "gamma"
      # "phi"
      # "cheating with amplitude here"
      n220 = Unbundle By Name(w401) -> ("normalization factor"=w400:dbl)
      n221 = Unbundle By Name(w385) -> ("z center"=w404:cdb, "z(inf)"=w403:cdb)
      n222 = Subtract(x=w404, y=w403) -> (x-y=w391:cdb)
      n223 = Add(x=w391, y=w404) -> (x+y=w390:cdb)
      n224 = Subtract(x=w390, y=w404) -> (x-y=w399:cdb)
      n225 = Complex To Polar(r * e^(i*theta)=w399) -> (r=w392:dbl, theta=w397:dbl)
      n226 = Add(x=1.5707963267948966, y=w397) -> (x+y=w396:dbl)
      n227 = Unbundle By Name(w389) -> ("omega"=w387:dbl, "gamma"=w388:dbl)
      n228 = Multiply(x=w392, y=w388) -> (x*y=w394:dbl)
      n229 = Divide(x=w387, y=w388) -> (x/y=w395:dbl)
      n230 = Multiply(x=w394, y=w400) -> (x*y=w393:dbl)
      n231 = Bundle By Name(cluster=w386, "Amplitude"=w393, "omega(0)"=w387, "Gamma"=w388, "phase"=w396, "Q"=w395, "Norm  Ampl"=w394, "z (inf)"=w403, "4corners"=w385) -> (w402:T1)
    }
  }
  n232 = Bundle By Name(cluster=w10, "phase around center"=w9, "three points"=w8) -> (w7:T3)
  "parameters out  : center detection" <- w7
  "lorentzian out" <- w12
